vi "PositionEstimator.vi"(8 "error in (no error)":errorcluster, 11 "Angles In":dbl[](array[numeric])) -> (0 "error out":errorcluster, 3 "Positions Out":dbl[](array[numeric]))   [LabVIEW 2018, in "Motor_ReadAng.lvlib"]
doc: "Takes the two angles as inputs and provides estmates for the positions."
uses:
  Motor_ReadAng.lvlib
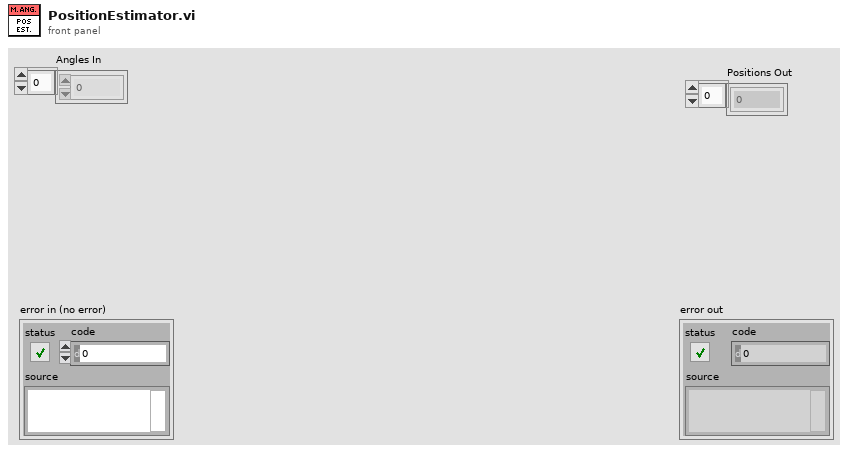
[diagram p1: front panel]
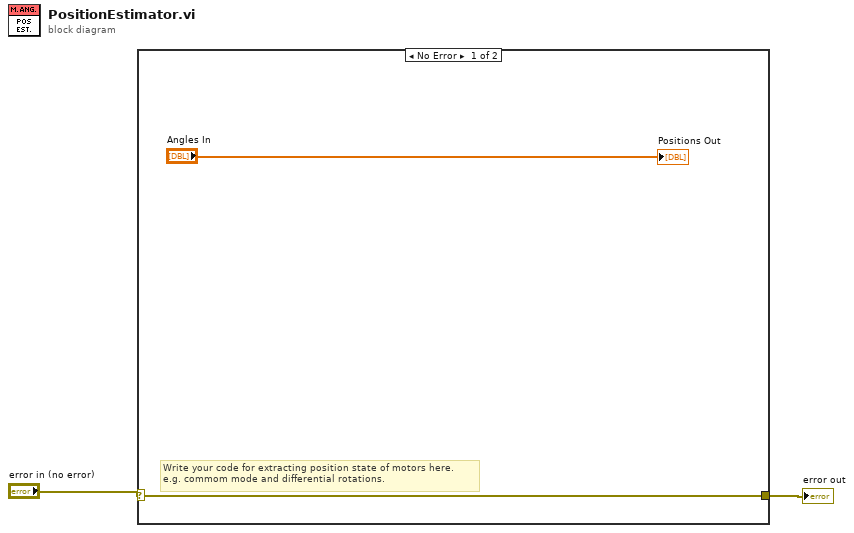
[diagram p0: block diagram]
diagram:
  n1 = case shown="No Error" "error in (no error)" {
    selector: "error in (no error)" -> [w4 w5]
    tunnel: [w4 w5] -> w1
    frame No Error {
      # "Write your code for extracting position state of motors here.\ne.g. commom mode and differential rotations."
      "Positions Out" <- "Angles In"
    }
    frame Error {
    }
  }
  "error out" <- w1
